vi "ReturnName.vi"(8 "error in (no error)":errorcluster, 11 "iClass in":refnum<class "iClass.lvclass">) -> (0 "error out":errorcluster, 2 "Name":string, 3 "iClass out":refnum<class "iClass.lvclass">)   [LabVIEW 2020, in "Mermaid.lvlib" / "iClass.lvclass"]
uses:
  iClass.lvclass
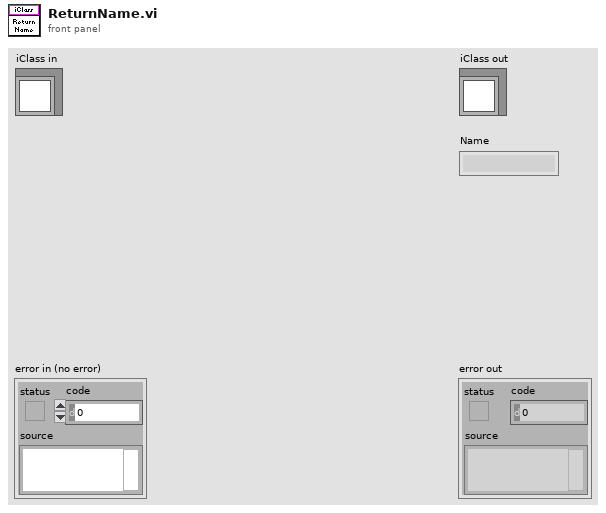
[diagram p1: front panel]
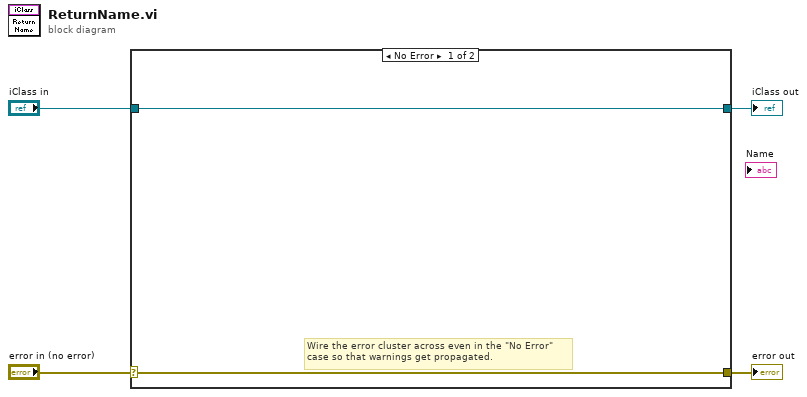
[diagram p0: block diagram]
diagram:
  n1 = case shown="No Error" "error in (no error)" {
    selector: "error in (no error)" -> [w5 w8]
    tunnel: [w5 w8] -> w3
    tunnel: [w6 w7] -> w1
    tunnel: "iClass in" -> [w6 w7]
    frame No Error {
      # "Wire the error cluster across even in the \"No Error\"\ncase so that warnings get propagated."
    }
    frame Error {
    }
  }
  "error out" <- w3
  "iClass out" <- w1
